vi "Extrapolate State.vi"(7 "Initial State":T1, 8 "G":T1, 9 "F":T1, 11 "Control":T1) -> (3 "Predicted State":T1)   [LabVIEW 2020]
uses:
  <vilib>/Analysis/Matrix/Datatypes/RealMatrix.ctl
  <vilib>/Analysis/baseanly.llb/Real A x B.vi
  <vilib>/Analysis/Matrix/Numeric/Add/Add - RM,RM.vi
  <vilib>/Analysis/NI_AALBase.lvlib
  <vilib>/Analysis/Matrix/NI_Matrix.lvlib
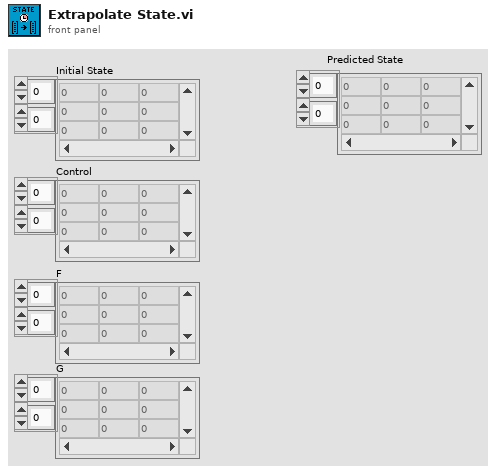
[diagram p1: front panel]
types:
  T1 = typedef "NI_Matrix.lvlib/RealMatrix.ctl" = dbl[][]
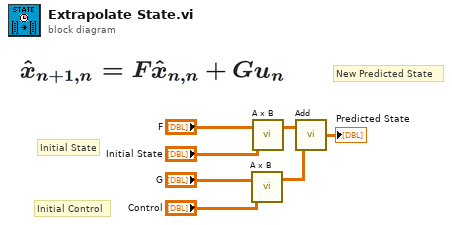
[diagram p0: block diagram]
diagram:
  # "Initial Control"
  # "Initial State"
  # "New Predicted State"
  n1 = call-poly <vilib>:"A x B.vi"("B"="Control", "A"="G") -> ("A x B"=w3:T1)  [unwired: 1 out]
  n2 = call-poly <vilib>:"A x B.vi"("B"="Initial State", "A"="F") -> ("A x B"=w2:T1)  [unwired: 1 out]
  n3 = call-poly <vilib>:"Add.vi"("Real Matrix B"=w3, "Real Matrix A"=w2) -> ("A + B"=→"Predicted State":T1)
